vi "GDSLvIcon_CreatePictureText.vi"(1 "Text":T1, 2 "Pixel width":i32=30, 3 "Max nr of rows":i32=3, 4 "Pixel height":i32=30, 5 "error in (no error)":errorcluster, 6 "Offset":cluster{"X":i32, "Y":i32}) -> (16 "CharPicture":bool[][](array[boolean]), 17 "X-Limited":bool, 18 "Y-Limited":bool, 19 "error out":errorcluster)   [LabVIEW 2020]
doc: "Creates a picture text based on the input string and optimize it for maximum pixel width and maximum number of rows."
uses:
  GDSLvIcon_TextDataType.ctl
  GDSLvIcon_WordCompressionType.ctl
  GDSLvIcon_TextAlignment.ctl
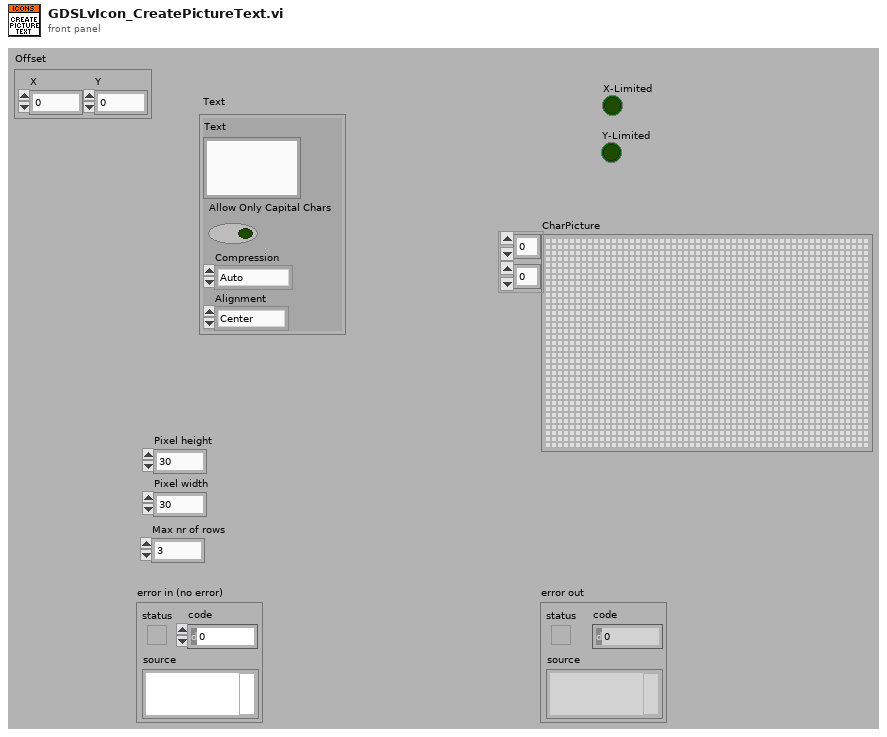
[diagram p1: front panel]
types:
  T1 = typedef "GDSLvIcon_TextDataType.ctl" = cluster{"Text":string, "Allow Only Capital Chars":bool, "Compression":T2, "Alignment":T3}
  T2 = typedef "GDSLvIcon_WordCompressionType.ctl" = enum16{"Auto", "On", "Off"}
  T3 = typedef "GDSLvIcon_TextAlignment.ctl" = enum16{"Center", "Left", "Right"}
  T4 = typedef "GDSLvIcon_WordDataType.ctl" = cluster{"WordPic":bool[][], "WordPic(Comp)":bool[][], "Width":i32, "Width(Comp)":i32, "Height":i32, "BaseOffset":i32}
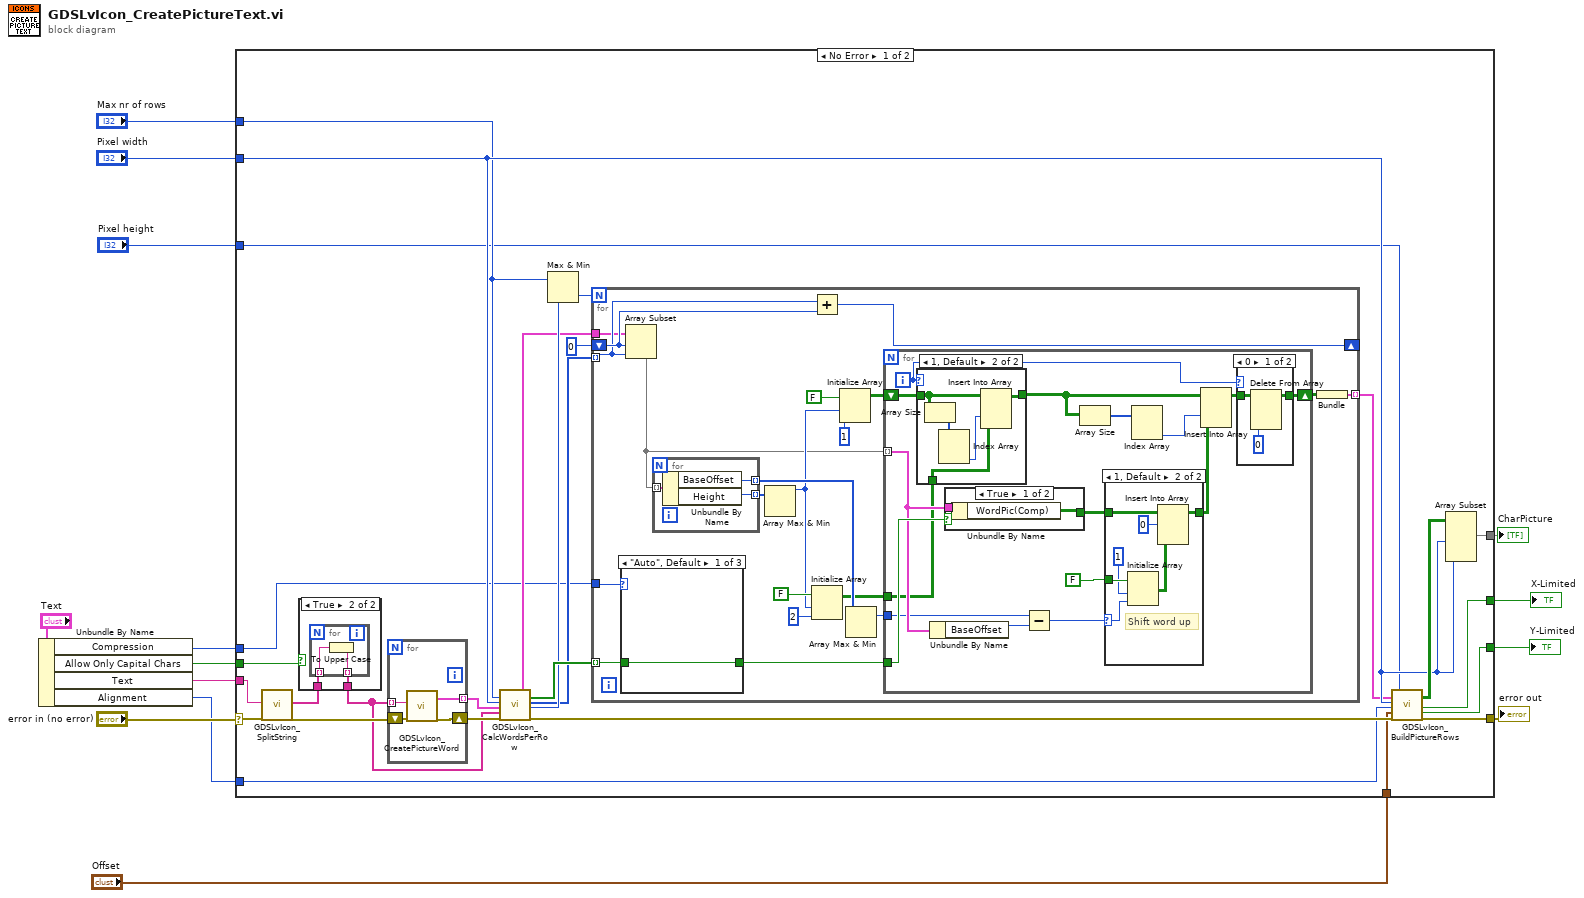
[diagram p0: block diagram]
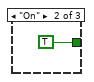
[diagram p3: hidden frame]
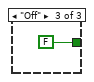
[diagram p4: hidden frame]
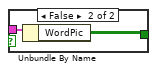
[diagram p8: hidden frame]
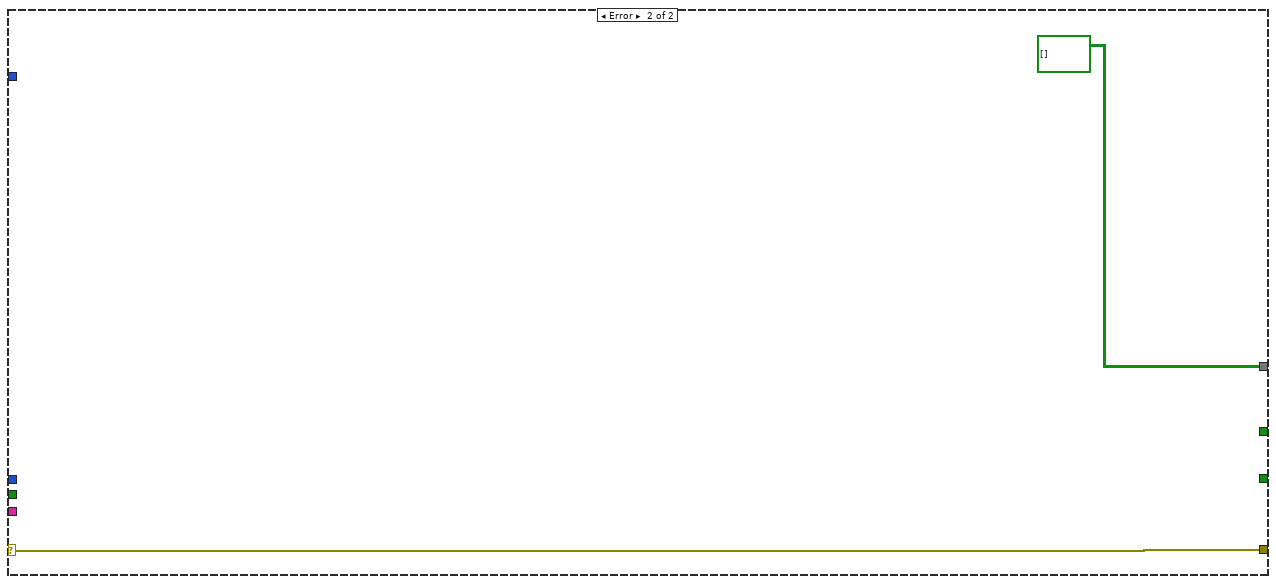
[diagram p9: hidden frame]
diagram:
  n1 = Unbundle By Name("Text") -> ("Compression"=w5:T2, "Allow Only Capital Chars"=w6:bool, "Text"=w7:string, "Alignment"=w4:T3)
  n2 = case shown="No Error" "error in (no error)" {
    selector: "error in (no error)" -> [w41 w116]
    tunnel: [w39 w116] -> w13
    tunnel: w7 -> [w40 _]
    tunnel: "Pixel width" -> [w33 _]
    tunnel: "Max nr of rows" -> [w31 _]
    tunnel: [w23 bool[][] [] ("CharPicture")] -> w9
    tunnel: "Pixel height" -> [w24 _]
    tunnel: w6 -> [w22 _]
    tunnel: w5 -> [w19 _]
    tunnel: w4 -> [w18 _]
    tunnel: "Offset" -> [w17 _]
    tunnel: [w16 _] -> w2
    tunnel: [w15 _] -> w1
    frame No Error {
      n3 = call "GDSLvIcon_SplitString.vi"("String"=w40, "error in (no error)"=w41) -> ("words"=w20:string[], "error out"=w37:errorcluster)  [unwired: 16 in]
      n4 = case shown="True" w22 {
        tunnel: w20 -> [w42 w44]
        tunnel: [w42 w43] -> w21
        frame False {
        }
        frame True {
          n5 = for {
            tunnel: w44 -> [w46] mode=indexing
            tunnel: [w45] -> w43 mode=indexing
            n6 = To Upper Case(1:w46) -> (0:w45:string)
          }
        }
      }
      n7 = for {
        tunnel: w21 -> [w114] mode=indexing
        shift-right: [w112] -> w36
        shift-left: w37 -> [w113]
        tunnel: [w111] -> w25 mode=indexing
        n8 = call "GDSLvIcon_CreatePictureWord.vi"("Word"=w114, "error in (no error)"=w113) -> ("WordData"=w111:T4, "error out"=w112:errorcluster)  [unwired: 16 in]
      }
      n9 = call "GDSLvIcon_CalcWordsPerRow.vi"("Max nr of rows"=w31, "Pixel width"=w33, "wordData"=w25, "words"=w21, "error in (no error)"=w36) -> ("wordData out"=w26:T4[], "CompressRow"=w34:bool[], "WordsPerRow"=w29:i32[], "NoOfRowsRequired"=w32:i32, "error out"=w35:errorcluster)  [unwired: 10 in]
      n10 = Max & Min(x=w31, y=w32) -> (min(x,y)=w30:i32)  [unwired: 1 out]
      n11 = for {
        N: w30 -> [_]
        tunnel: w26 -> [w59]
        tunnel: w29 -> [w65] mode=indexing
        shift-right: [w64] -> _
        shift-left: 0 -> [w66]
        tunnel: w34 -> [w48] mode=indexing
        tunnel: [w62] -> w27 mode=indexing
        tunnel: w19 -> [w49]
        n12 = case shown="\"Auto\", Default" w49 {
          tunnel: w48 -> [w67 _ _]
          tunnel: [w67 TRUE FALSE] -> w47
          frame "Auto", Default {
          }
          frame "On" {
          }
          frame "Off" {
          }
        }
        n13 = Array Subset(array=w59, index=w66, length=w65) -> (w51:T4[])
        n14 = for {
          tunnel: w51 -> [w72] mode=indexing
          tunnel: [w71] -> w58 mode=indexing
          tunnel: [w70] -> w57 mode=indexing
          n15 = Unbundle By Name(w72) -> ("BaseOffset"=w70:i32, "Height"=w71:i32)
        }
        n16 = Array Max & Min(array=w58) -> (max value=w52:i32)  [unwired: 3 out]
        n17 = Add(x=w66, y=w65) -> (x+y=w64:i32)
        n18 = Initialize Array(FALSE, w52, 2 ("Dimension Size")) -> (w53:bool[][])
        n19 = Initialize Array(FALSE, w52, 1 ("Numeric")) -> (w63:bool[][])
        n20 = Array Max & Min(array=w57) -> (max value=w56:i32)  [unwired: 3 out]
        n21 = for {
          tunnel: w51 -> [w83] mode=indexing
          tunnel: w47 -> [w88]
          shift-right: [w75] -> w60
          shift-left: w63 -> [w87]
          tunnel: w56 -> [w80]
          tunnel: w53 -> [w77]
          i -> [w73]
          n22 = case shown="1, Default" w73 {
            tunnel: [w101 w106] -> w86
            tunnel: w87 -> [w101 w105]
            tunnel: w77 -> [_ w102]
            frame 0 {
            }
            frame 1, Default {
              n23 = Array Size(array=w105) -> (size(s)=w104:i32[])
              n24 = Index Array(array=w104) -> (element #2=w103:i32)  [unwired: 2 in, 1 out]
              n25 = Insert Into Array(array=w105, index (col)=w103, new element=w102) -> (w106:bool[][])  [unwired: 1 in]
            }
          }
          n26 = Unbundle By Name(w83) -> ("BaseOffset"=w79:i32)
          n27 = case shown="True" w88 {
            tunnel: w83 -> [w108 w110]
            tunnel: [w107 w109] -> w82
            frame True {
              n28 = Unbundle By Name(w108) -> ("WordPic(Comp)"=w107:bool[][])
            }
            frame False {
              n29 = Unbundle By Name(w110) -> ("WordPic"=w109:bool[][])
            }
          }
          n30 = Subtract(x=w80, y=w79) -> (x-y=w78:i32)
          n31 = Array Size(array=w86) -> (size(s)=w85:i32[])
          n32 = case shown="1, Default" w78 {
            selector: w78 -> [_ w94]
            tunnel: w82 -> [w93 w100]
            tunnel: [w93 w99] -> w81
            tunnel: FALSE -> [_ w98]
            frame 0 {
            }
            frame 1, Default {
              # "Shift word up"
              n33 = Initialize Array(w98, 1 ("Numeric"), w94) -> (w97:bool[][])
              n34 = Insert Into Array(array=w100, index (row)=0 ("Index (row)"), new element=w97) -> (w99:bool[][])  [unwired: 1 in]
            }
          }
          n35 = Index Array(array=w85) -> (element #2=w84:i32)  [unwired: 2 in, 1 out]
          n36 = Insert Into Array(array=w86, index (col)=w84, new element=w81) -> (w74:bool[][])  [unwired: 1 in]
          n37 = case shown="0" w73 {
            tunnel: [w89 w92] -> w75
            tunnel: w74 -> [w91 w92]
            frame 0 {
              n38 = Delete From Array(array=w91, index (col)=0 ("Disabled Index (col)")) -> (array with subset deleted=w89:bool[][])  [unwired: 2 in, 1 out]
            }
            frame Default {
            }
          }
        }
        n39 = Bundle(w60) -> (w62:cluster{bool[][]})  [unwired: 1 in]
      }
      n40 = call "GDSLvIcon_BuildPictureRows.vi"("RowTextPictures"=w27, "Pixel width"=w33, "Alignment"=w18, "Offset"=w17, "error in (no error)"=w35, "Pixel height"=w24) -> ("CharPicture"=w38:bool[][], "X-Limited"=w16:bool, "Y-Limited"=w15:bool, "error out"=w39:errorcluster)  [unwired: 10 in]
      n41 = Array Subset(array=w38, length (row)=w33, length (col)=w33) -> (w23:bool[][])  [unwired: 2 in]
    }
    frame Error {
    }
  }
  "error out" <- w13
  "CharPicture" <- w9
  "Y-Limited" <- w1
  "X-Limited" <- w2
